vi "TDV_TESTING_GenerateSweepFolders.vi"(6 "base path":path, 7 "SuperSweep ID":string, 8 "Supersweep step Size":dbl format="%#_13g", 9 "Supersweep end Value":dbl format="%#_13g", 10 "Supersweep start Value":dbl format="%#_13g", 11 "Subsweep Identifier":string) -> ()   [LabVIEW 2016]
uses:
  METADATA.ctl
  <vilib>/regexp/Match Regular Expression.xnode
panel:
  in  "Comments":string
  in  "Terminal Info Clusters":T1(array[cluster])=[{"Terminal Identifier"="28-SG1", "AC Freq"=0.0, "AC Amp"=0.0, "DC Amp"=0.0}]
  in  "Metadata Cluster":T2
  # "Ex:\nSupersweep: BG\nSubsweep: SG1"
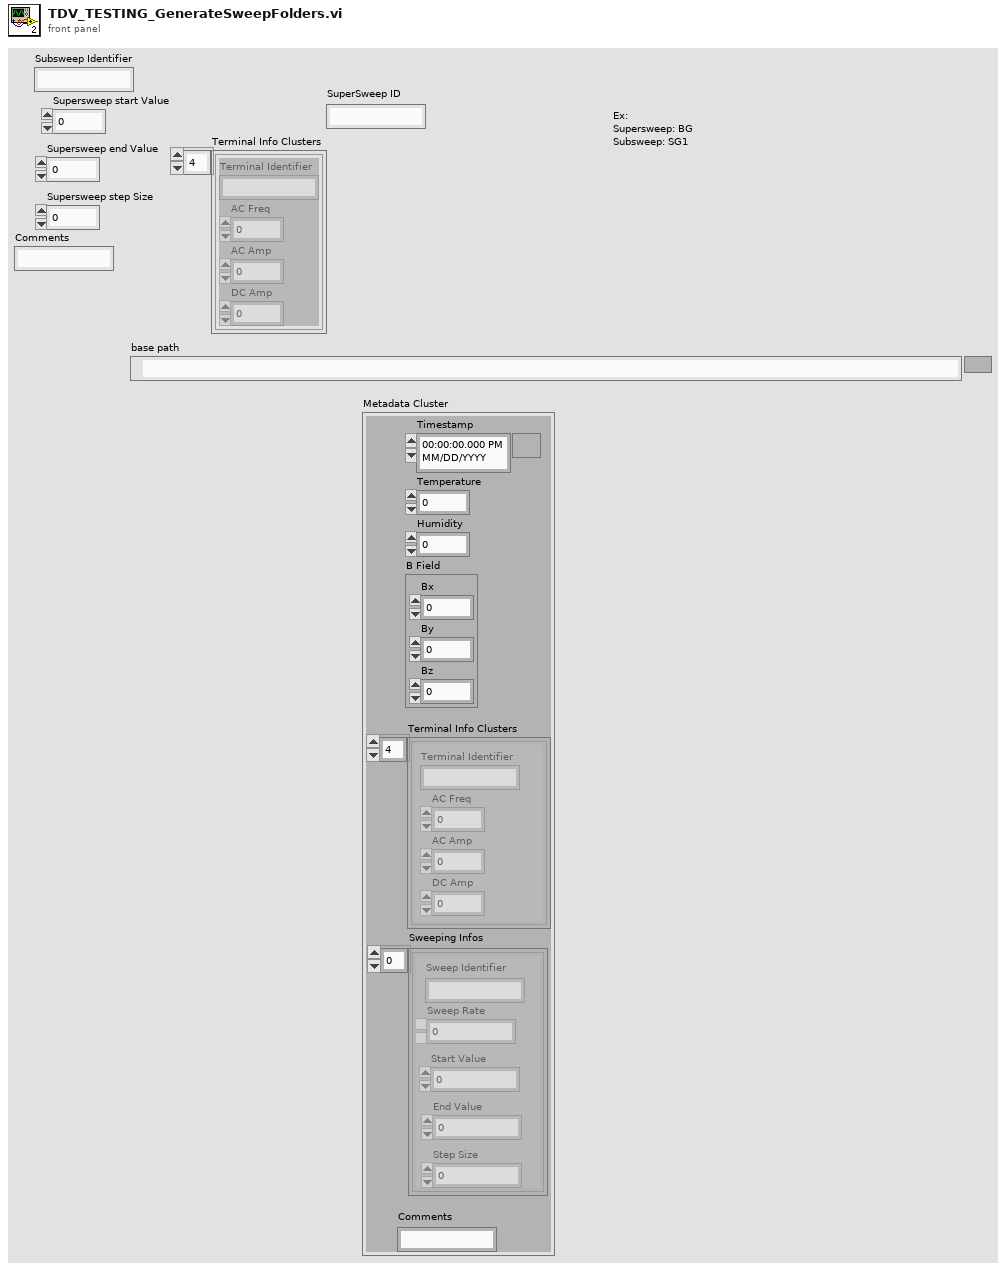
[diagram p1: front panel]
types:
  T1 = cluster{"Terminal Identifier":string, "AC Freq":dbl, "AC Amp":dbl, "DC Amp":dbl}[]
  T2 = typedef "METADATA.ctl" = cluster{"Timestamp":timestamp, "Temperature":dbl, "Humidity":dbl, "B Field":cluster{"Bx":dbl, "By":dbl, "Bz":dbl}, "Terminal Info Clusters":cluster{"Terminal Identifier":string, "AC Freq":dbl, "AC Amp":dbl, "DC Amp":dbl}[], "Sweeping Infos":cluster{"Sweep Rate":dbl, "Sweep Identifier":string, "Start Value":dbl, "End Value":dbl, "Step Size":dbl}[], "Comments":string}
  T3 = cluster{"Sweep Rate":dbl, "Sweep Identifier":string, "Start Value":dbl, "End Value":dbl, "Step Size":dbl}[]
  T4 = cluster{"Sweep Rate":dbl, "Sweep Identifier":string, "Start Value":dbl, "End Value":dbl, "Step Size":dbl}
  T5 = cluster{"Terminal Identifier":string, "AC Freq":dbl, "AC Amp":dbl, "DC Amp":dbl}
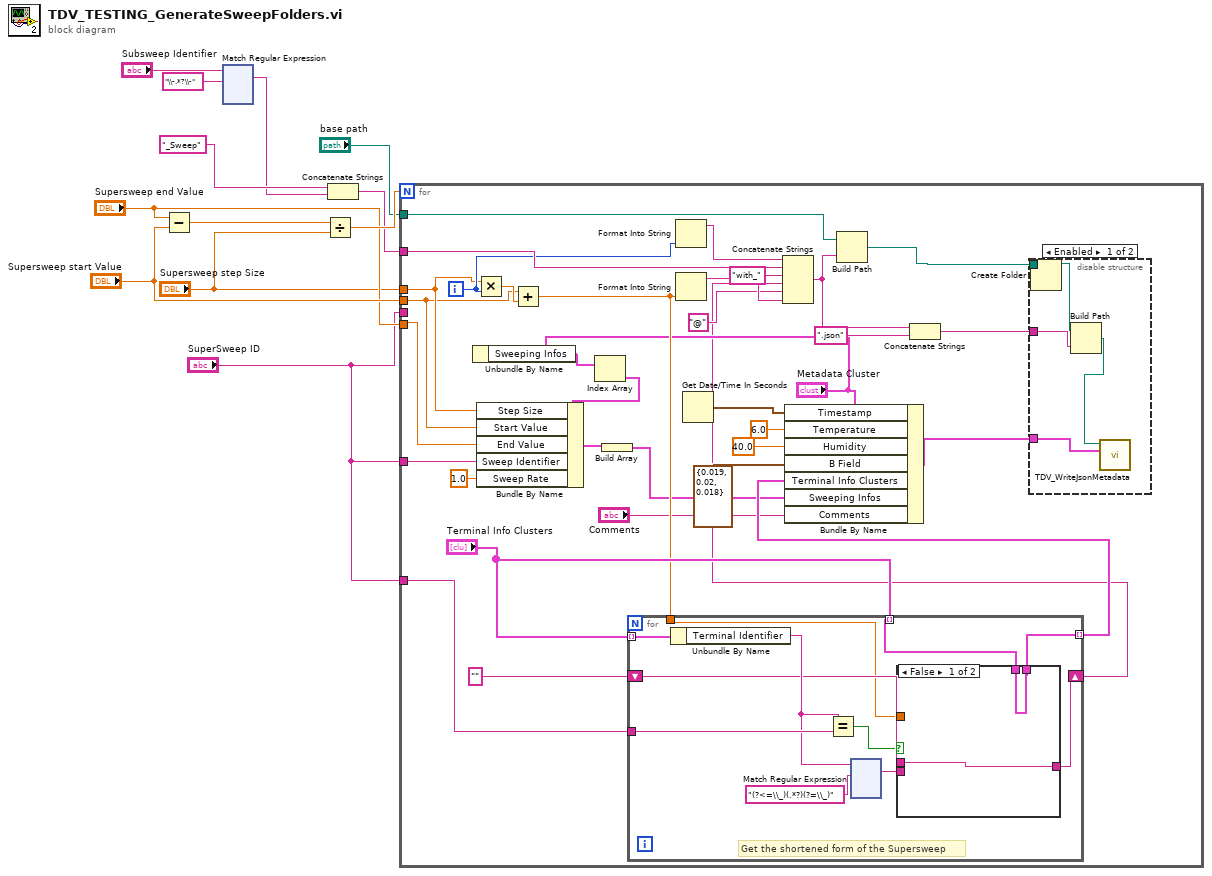
[diagram p0: block diagram]
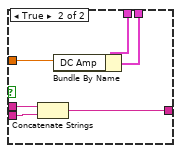
[diagram p3: hidden frame]
diagram:
  n1 = Subtract(x="Supersweep end Value", y="Supersweep start Value") -> (x-y=w12:dbl)
  n2 = xnode "Match Regular Expression"("input string"="Subsweep Identifier", "regular expression"="\\-.*?\\-") -> ("whole match"=w2:string)  [unwired: 4 in, 4 out]
  n3 = Divide(x=w12, y="Supersweep step Size") -> (x/y=w11:dbl)
  n4 = Concatenate Strings("_Sweep" ("string"), w2) -> (w6:string)
  n5 = for {
    N: w11 -> [_]
    tunnel: "base path" -> [w46]
    tunnel: "Supersweep start Value" -> [w20]
    tunnel: "Supersweep end Value" -> [w19]
    tunnel: "Supersweep step Size" -> [w24]
    tunnel: "SuperSweep ID" -> [_]
    tunnel: w6 -> [w44]
    tunnel: "SuperSweep ID" -> [w29]
    tunnel: "SuperSweep ID" -> [w18]
    i -> [w42]
    n6 = Unbundle By Name("Metadata Cluster") -> ("Sweeping Infos"=w22:T3)
    n7 = Multiply(x=w24, y=w42) -> (x*y=w45:dbl)
    n8 = Add(x=w20, y=w45) -> (x+y=w26:dbl)
    n9 = Index Array(array=w22) -> (element=w21:T4)  [unwired: 1 in]
    n10 = Bundle By Name(cluster=w21, "Step Size"=w24, "Start Value"=w20, "End Value"=w19, "Sweep Identifier"=w18, "Sweep Rate"=1.0) -> (w16:T4)
    n11 = Build Array(w16) -> (w15:T3)
    n12 = for {
      tunnel: "Terminal Info Clusters" -> [w62] mode=indexing
      tunnel: w29 -> [w61]
      shift-right: [w55] -> w13
      shift-left: "" -> [w57]
      tunnel: "Terminal Info Clusters" -> [w54] mode=indexing
      tunnel: w26 -> [w53]
      tunnel: [w52] -> w25 mode=indexing
      # "Get the shortened form of the Supersweep"
      n13 = Unbundle By Name(w62) -> ("Terminal Identifier"=w60:string)
      n14 = Equal?(x=w60, y=w61) -> (x = y?=w56:bool)
      n15 = xnode "Match Regular Expression"("input string"=w60, "regular expression"="(?<=\\_)(.*?)(?=\\_)") -> ("whole match"=w58:string)  [unwired: 4 in, 4 out]
      n16 = case shown="False" w56 {
        tunnel: w58 -> [_ w70]
        tunnel: w57 -> [w64 w69]
        tunnel: [w64 w68] -> w55
        tunnel: w54 -> [w63 w67]
        tunnel: w53 -> [_ w66]
        tunnel: [w63 w65] -> w52
        frame False {
        }
        frame True {
          n17 = Concatenate Strings(w69, w70) -> (w68:string)
          n18 = Bundle By Name(cluster=w67, "DC Amp"=w66) -> (w65:T5)
        }
      }
    }
    n19 = Format Into String(w42) -> (resulting string=w41:string)  [unwired: 3 in, 1 out]
    n20 = Format Into String(w26) -> (resulting string=w40:string)  [unwired: 3 in, 1 out]
    n21 = Get Date/Time In Seconds() -> (seconds since 1Jan1904=w34:timestamp)
    n22 = Concatenate Strings(w41, w44, "with_" ("string"), w13, "@" ("string"), w40) -> (w37:string)
    n23 = Bundle By Name(cluster="Metadata Cluster", "Timestamp"=w34, "Temperature"=6.0, "Humidity"=40.0, "B Field"=cluster{"Bx":dbl, "By":dbl, "Bz":dbl} {"Bx"=0.019, "By"=0.02, "Bz"=0.018}, "Terminal Info Clusters"=w25, "Sweeping Infos"=w15, "Comments"="Comments") -> (w30:T2)
    n24 = Build Path(base path=w46, name or relative path=w37) -> (appended path=w43:path)
    n25 = Concatenate Strings(w37, ".json" ("string")) -> (w35:string)
    n26 = disable-structure shown="Enabled" {
      disable-tunnel: w43 -> [w51 _]
      disable-tunnel: w35 -> [w49 _]
      disable-tunnel: w30 -> [w47 _]
      frame Enabled {
        n27 = Create Folder(path (use dialog)=w51) -> (created path=w50:path)  [unwired: 2 in, 2 out]
        n28 = Build Path(base path=w50, name or relative path=w49) -> (appended path=w48:path)
        n29 = call "TDV_WriteJsonMetadata.vi"("Metadata Cluster"=w47, "JSON destination"=w48) -> ()  [unwired: 6 in, 4 out]
      }
      frame Disabled {
      }
    }
  }
